vi "Close.vi"(8 "Error In":errorcluster, 11 "Hue Config":T1) -> (0 "Error Out":errorcluster)   [LabVIEW 2013, in "LVH-Hue.lvlib"]
uses:
  LVH-Hue.lvlib
  Private/Type Defs/Hue Ref.ctl
  <vilib>/httpClient/ClientHandle.ctl
  Private/Type Defs/Light.ctl
  <vilib>/httpClient/LabVIEWHTTPClient.lvlib
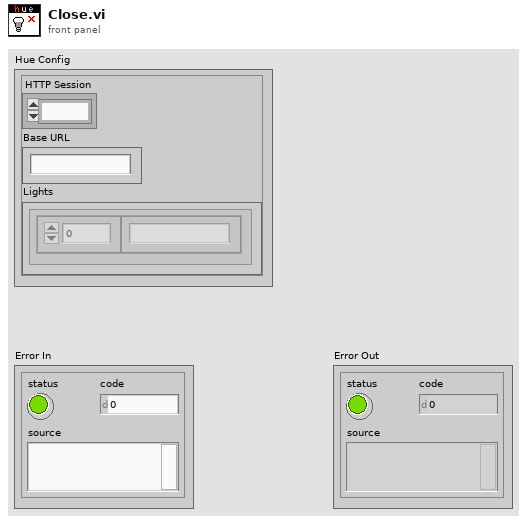
[diagram p1: front panel]
types:
  T1 = typedef "LVH-Hue.lvlib/Hue Ref.ctl" = cluster{"HTTP Session":T2, "Base URL":string, "Lights":T3[]}
  T2 = typedef "LabVIEWHTTPClient.lvlib/ClientHandle.ctl" = refnum<k1>
  T3 = typedef "LVH-Hue.lvlib/Light.ctl" = cluster{"ID":i32, "Name":string}
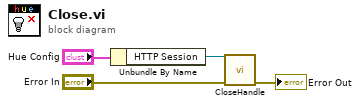
[diagram p0: block diagram]
diagram:
  n1 = Unbundle By Name("Hue Config") -> ("HTTP Session"=w3:T2)
  n2 = call <vilib>:"CloseHandle.vi"("client handle"=w3, "error in (no error)"="Error In") -> ("error out"=→"Error Out":errorcluster)  [unwired: 13 in]
